vi "DSF.Engine.Execution.Framework.Initialize Cache.vi"(8 "error in (no error)":errorcluster, 11 "Framework in":refnum<class "DSF.Engine.Execution.Framework.lvclass">) -> (0 "error out":errorcluster, 3 "Framework out":refnum<class "DSF.Engine.Execution.Framework.lvclass">)   [LabVIEW 2016, in "DSF.Engine.lvlib" / "DSF.Engine.Execution.Framework.lvclass"]
uses:
  DSF.Engine.Execution.Framework.lvclass
  Cache/DSF.Engine.Memory.Cache.Framework.lvclass
  DSF.Engine.Execution.Framework.lvclass/DSF.Engine.Execution.Framework.ctl
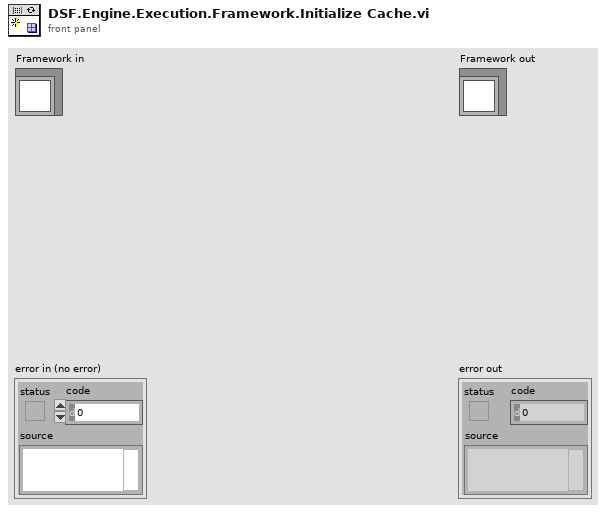
[diagram p1: front panel]
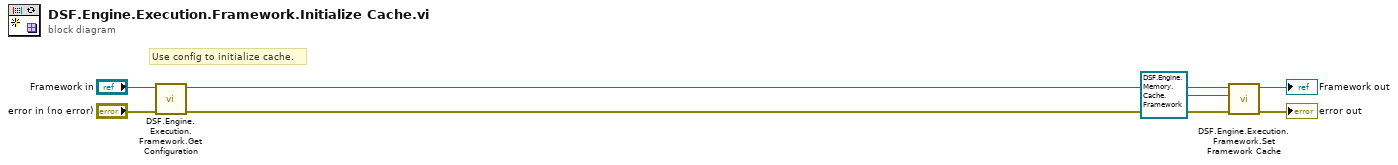
[diagram p0: block diagram]
diagram:
  # "Use config to initialize cache."
  n1 = call "DSF.Engine.Execution.Framework.Get Configuration.vi"("error in (no error)"="error in (no error)", "Framework in"="Framework in") -> ("error out"=w2:errorcluster, "Framework out"=w5:refnum<class "DSF.Engine.Execution.Framework.lvclass">)  [unwired: 7 in, 1 out]
  n2 = call "DSF.Engine.Execution.Framework.Set Framework Cache.vi"("error in (no error)"=w2, "Framework Cache"=refnum<class "DSF.Engine.Memory.Cache.Framework.lvclass"> refnum, "Framework in"=w5) -> ("error out"=→"error out":errorcluster, "Framework out"=→"Framework out":refnum<class "DSF.Engine.Execution.Framework.lvclass">)  [unwired: 7 in]
